vi "Copy Linked List.vi"(4 "New Linked List ID":string, 5 "Recursive? (T)":bool=TRUE, 6 "Move?":bool, 7 "New Parent Linked List ID":string, 8 "error in (no error)":errorcluster, 9 "Insertion Index":i32=-1, 10 "Linked List ID":string, 11 "Linked List Ref":refnum<data-value>) -> (0 "error out":errorcluster, 1 "Children IDs out":string[](array[string]), 2 "Linked List ID out":string, 3 "Linked List Ref out":refnum<data-value>)   [LabVIEW 2020, in "Linked Lists.lvlib" / "Linked List Ref.lvclass"]
uses:
  <vilib>/gpm_packages/@cs/linked-list/Source/Linked List/Linked List Ref/Linked List Ref.lvclass
  <vilib>/gpm_packages/@cs/linked-list/Source/Linked List/ILinkedList/ILinked List.lvclass
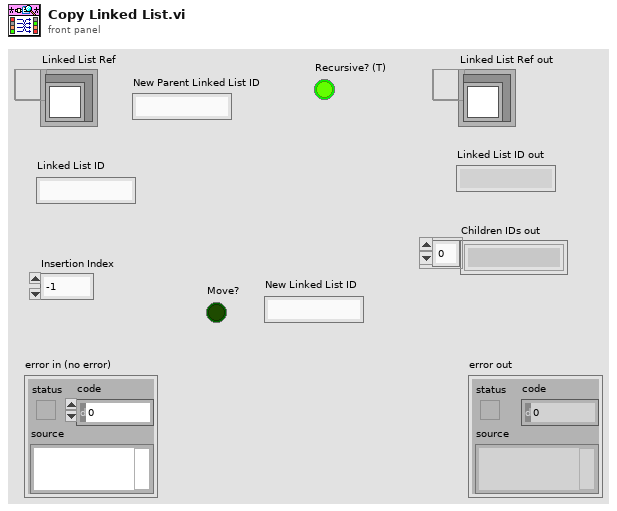
[diagram p1: front panel]
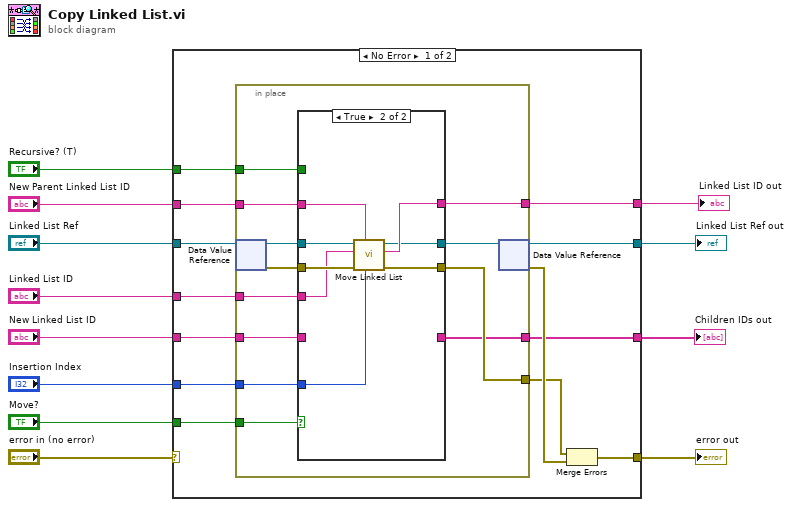
[diagram p0: block diagram]
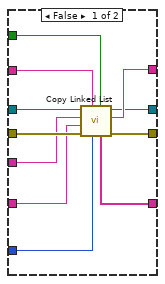
[diagram p2: hidden frame]
diagram:
  n1 = case shown="No Error" "error in (no error)" {
    selector: "error in (no error)" -> [_ w58]
    tunnel: "Linked List Ref" -> [w25 w57]
    tunnel: "New Parent Linked List ID" -> [w24 _]
    tunnel: "Linked List ID" -> [w23 _]
    tunnel: [w21 w58] -> w8
    tunnel: [w22 w57] -> w7
    tunnel: "Move?" -> [w19 _]
    tunnel: "Insertion Index" -> [w18 _]
    tunnel: "New Linked List ID" -> [w16 _]
    tunnel: [w15 _] -> w3
    tunnel: [w14 _] -> w2
    tunnel: "Recursive? (T)" -> [w13 _]
    frame No Error {
      n2 = in-place {
        in-place-border: w24 -> [w35]
        in-place-border: w23 -> [w31]
        in-place-border: w19 -> [w28]
        in-place-border: w18 -> [w34]
        in-place-border: [w29] -> w17
        in-place-border: w16 -> [w33]
        in-place-border: [w32] -> w15
        in-place-border: [w27] -> w14
        in-place-border: w13 -> [w26]
        n3 = in-place-dvr #1(w25) -> (w37:refnum<class "ILinked List.lvclass">, w36:errorcluster)
        n4 = case shown="True" w28 {
          tunnel: w37 -> [w48 w56]
          tunnel: w36 -> [w47 w51]
          tunnel: w35 -> [w46 w55]
          tunnel: w34 -> [w45 w50]
          tunnel: w33 -> [w44 _]
          tunnel: [w43 w54] -> w32
          tunnel: w31 -> [w42 w49]
          tunnel: [w41 w53] -> w30
          tunnel: [w40 w52] -> w29
          tunnel: [w39 _] -> w27
          tunnel: w26 -> [w38 _]
          frame False {
            n5 = call-dynamic "Copy Linked List.vi"("Recursive? (T)"=w38, "Insertion Index"=w45, "New Parent Linked List ID"=w46, "error in (no error)"=w47, "New Linked List ID"=w44, "Linked List ID"=w42, "ILinked List in"=w48) -> ("error out"=w40:errorcluster, "Linked List ID out"=w43:string, "ILinked List out"=w41:refnum<class "ILinked List.lvclass">, "Children"=w39:string[])  [unwired: 1 in]
          }
          frame True {
            n6 = call-dynamic "Move Linked List.vi"("Insertion Index"=w50, "New Parent Linked List ID"=w55, "error in (no error)"=w51, "Linked List ID"=w49, "ILinked List in"=w56) -> ("error out"=w52:errorcluster, "Linked List ID out"=w54:string, "ILinked List out"=w53:refnum<class "ILinked List.lvclass">)  [unwired: 4 in]
          }
        }
        n7 = in-place-dvr #1(w30) -> (w22:refnum<data-value>, w20:errorcluster)
      }
      n8 = Merge Errors(w17, w20) -> (w21:errorcluster)
    }
    frame Error {
    }
  }
  "error out" <- w8
  "Linked List Ref out" <- w7
  "Linked List ID out" <- w3
  "Children IDs out" <- w2
